vi "GetText.vi"(8 "error in":errorcluster, 11 "Engine in":refnum<class "Engine Parent Editor Node.lvclass">) -> (0 "error out":errorcluster, 1 "additional text":string, 2 "text":string, 3 "Engine out":refnum<class "Engine Parent Editor Node.lvclass">, 4 "glyph":string)   [LabVIEW 2013, in "PL Framework Configuration Tool.lvlib" / "Engine Parent Editor Node.lvclass"]
uses:
  Engine Parent Editor Node.lvclass
  subVIs/Glyphs Status.ctl
  <vilib>/NI/Configuration Framework/serializable configuration/get alias.vi
  PL Framework Configuration Tool.lvlib
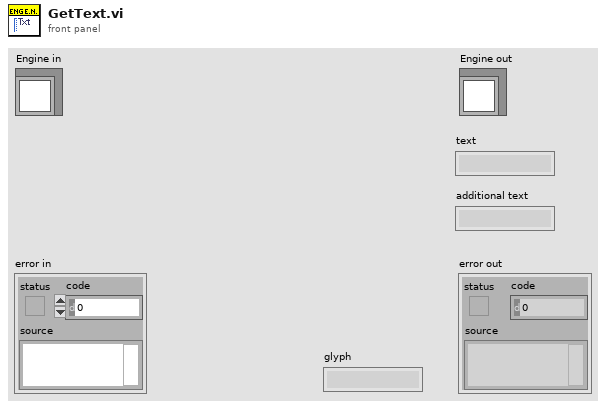
[diagram p1: front panel]
types:
  T1 = typedef "PL Framework Configuration Tool.lvlib/Glyphs Status.ctl" = enum16{"Normal", "Error"}
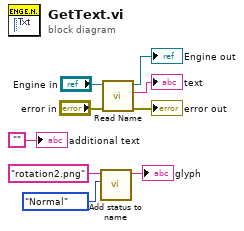
[diagram p0: block diagram]
diagram:
  n1 = call "Add status to name.vi"("Status"=Glyphs_Status."Normal", "Name"="rotation2.png" ("glyph")) -> ("Name with status"=→"glyph":string)  [unwired: 9 in]
  n2 = call "Read Name.vi"("error in"="error in", "Engine in"="Engine in") -> ("error out"=→"error out":errorcluster, "Name"=→"text":string, "Engine out"=→"Engine out":refnum<class "Engine Parent Editor Node.lvclass">)  [unwired: 7 in]
  "additional text" <- ""
